vi "Model.vi"(9 "th":dbl, 10 "wl":dbl, 11 "wr":dbl) -> (1 "thd":dbl, 2 "yd":dbl, 3 "xd":dbl)   [LabVIEW 2017]
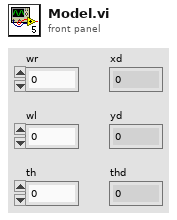
[diagram p1: front panel]
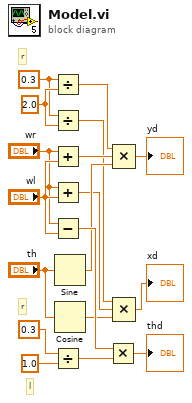
[diagram p0: block diagram]
diagram:
  w15 = 2.0 ("y")
  w14 = 0.3
  # "l"
  # "r"
  # "r"
  n1 = Divide(x=w14, y=w15) -> (x/y=w6:dbl)
  n2 = Divide(x=w14, y=w15) -> (x/y=w3:dbl)
  n3 = Add(x="wr", y="wl") -> (x+y=w7:dbl)
  n4 = Add(x="wr", y="wl") -> (x+y=w4:dbl)
  n5 = Subtract(x="wr", y="wl") -> (x-y=w13:dbl)
  n6 = Divide(x=0.3, y=1.0) -> (x/y=w12:dbl)
  n7 = Sine(x="th") -> (sin(x)=w8:dbl)
  n8 = Cosine(x="th") -> (cos(x)=w5:dbl)
  n9 = Multiply(x=w13, y=w12) -> (x*y=→"thd":dbl)
  n10 = Compound Arithmetic op=MULTIPLY(w6, w7, w8) -> (→"yd":dbl)
  n11 = Compound Arithmetic op=MULTIPLY(w3, w4, w5) -> (→"xd":dbl)
